vi "Rinocloud_get_metadata_field_value.vi"(6 "id":string, 9 "JSON Tree Expanded Reference":refnum<vi>) -> (0 "Notes":string, 1 "Tags":string, 2 "Name":string, 3 "Tree Ref out":refnum<vi>, 4 "body":string, 5 "headers":string)   [LabVIEW 2013]
uses:
  Rinocloud_global_variable.vi
  <vilib>/httpClient/POSTBuffer.vi
  <vilib>/LVH/i3 JSON/JSON Parsing/Get Object Parameter Files/Get Object Parameter - String.vi
  <vilib>/LVH/i3 JSON/JSON Parsing/Get Object Parameter Files/Get Object Parameter - Array.vi
  <vilib>/LVH/i3 JSON/JSON Parsing/Get Array Value at Index Files/Get Array Value at Index - String.vi
  <vilib>/httpClient/LabVIEWHTTPClient.lvlib
  i3 JSON/i3-json.lvlib
panel:
  out "JSON Tree":variant
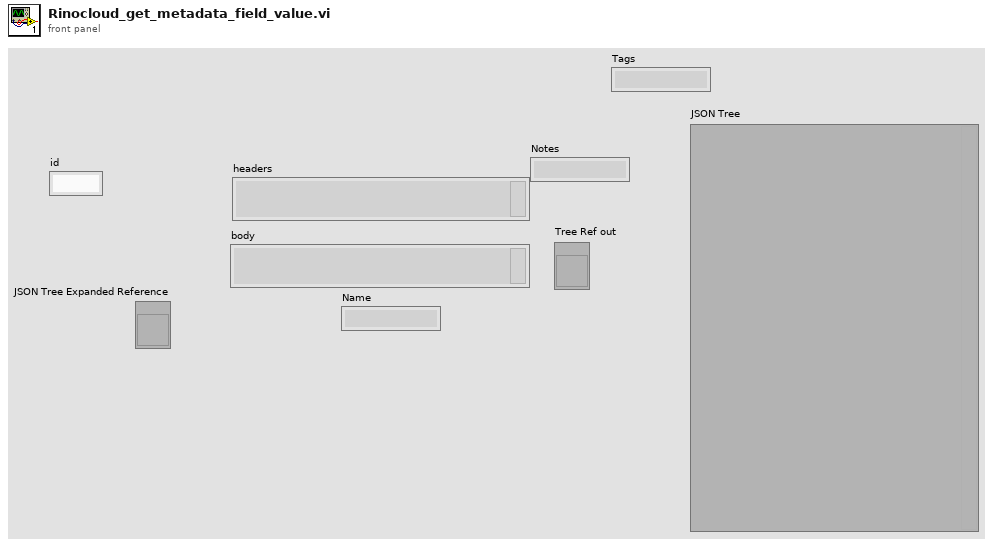
[diagram p1: front panel]
types:
  T1 = typedef "LabVIEWHTTPClient.lvlib/ClientHandle.ctl" = refnum<k1>
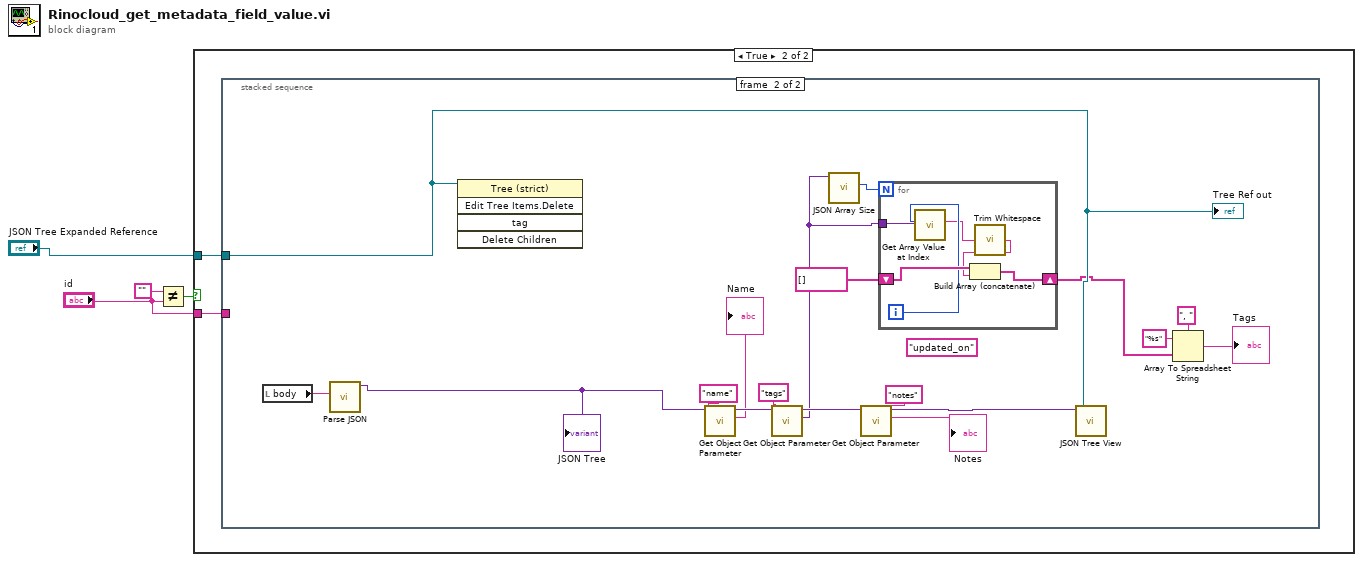
[diagram p0: block diagram]
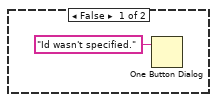
[diagram p2: hidden frame]
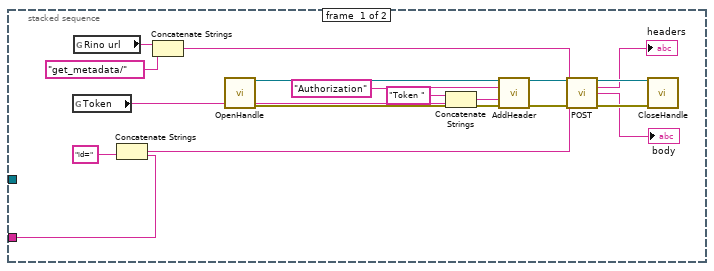
[diagram p3: hidden frame]
diagram:
  n1 = Not Equal?(x="", y="id") -> (x != y?=w3:bool)
  n2 = case shown="True" w3 {
    tunnel: "JSON Tree Expanded Reference" -> [_ w7]
    tunnel: "id" -> [_ w6]
    frame False {
      n3 = One Button Dialog(message="Id wasn't specified.") -> ()  [unwired: 1 in, 1 out]
    }
    frame True {
      n4 = stacked-sequence {
        tunnel: w7 -> [_ w34]
        tunnel: w6 -> [w9 _]
        frame #0 {
          n5 = global read "Rinocloud_global_variable.vi" "Token"() -> (w17:string)
          n6 = global read "Rinocloud_global_variable.vi" "Rino url"() -> (w23:string)
          n7 = Concatenate Strings("id=" ("value"), w9) -> (w8:string)
          n8 = Concatenate Strings(w23, "get_metadata/" ("Combo Box 2")) -> (w25:string)
          n9 = call <vilib>:"OpenHandle.vi"() -> ("client handle out"=w21:T1, "error out"=w18:errorcluster)  [unwired: 14 in]
          n10 = Concatenate Strings("Token " ("value"), w17) -> (w19:string)
          n11 = call <vilib>:"AddHeader.vi"("client handle"=w21, "header"="Authorization" ("url"), "value"=w19, "error in (no error)"=w18) -> ("client handle out"=w14:T1, "error out"=w13:errorcluster)  [unwired: 10 in]
          n12 = call-poly <vilib>:"POST.vi"("client handle"=w14, "url"=w25, "buffer"=w8, "error in (no error)"=w13) -> ("client handle out"=w16:T1, "headers"=→"headers":string, "body"=→"body":string, "error out"=w15:errorcluster)  [unwired: 8 in]
          n13 = call <vilib>:"CloseHandle.vi"("client handle"=w16, "error in (no error)"=w15) -> ()  [unwired: 13 in, 1 out]
        }
        frame #1 {
          (unwired) "updated_on" ("Parameter Name")
          n14 = local read "body"() -> (w43:string)
          n15 = call <vilib>:"Parse JSON.vi"("JSON String"=w43) -> ("JSON Tree"=w33:variant)  [unwired: 7 in, 3 out]
          "JSON Tree" <- w33
          n16 = invoke class="Tree (strict)" method="Edit Tree Items.Delete"(reference=w34) -> ()  [unwired: 4 in, 5 out]
          n17 = call-poly <vilib>:"Get Object Parameter.vi"("Parameter Name"="name", "JSON Tree In (JSON Object)"=w33) -> ("String Value"=→"Name":string, "JSON Tree Out Passthrough"=w40:variant)  [unwired: 6 in, 2 out]
          n18 = call-poly <vilib>:"Get Object Parameter.vi"("Parameter Name"="tags", "JSON Tree In (JSON Object)"=w40) -> ("JSON Array"=w31:variant, "JSON Tree Out Passthrough"=w38:variant)  [unwired: 6 in, 2 out]
          n19 = call <vilib>:"JSON Array Size.vi"("JSON Tree In (JSON Array)"=w31) -> ("Array Size"=w32:i32)  [unwired: 8 in, 2 out]
          n20 = call-poly <vilib>:"Get Object Parameter.vi"("Parameter Name"="notes", "JSON Tree In (JSON Object)"=w38) -> ("String Value"=→"Notes":string, "JSON Tree Out Passthrough"=w35:variant)  [unwired: 6 in, 2 out]
          n21 = for {
            N: w32 -> [_]
            tunnel: w31 -> [w49]
            shift-right: [w47] -> w27
            shift-left: string[] [] ("Tags 2") -> [w48]
            i -> [w46]
            n22 = call-poly <vilib>:"Get Array Value at Index.vi"("Index"=w46, "JSON Tree In (JSON Array)"=w49) -> ("String Value"=w45:string)  [unwired: 6 in, 3 out]
            n23 = call <vilib>:"Trim Whitespace.vi"("string"=w45) -> ("trimmed string"=w44:string)  [unwired: 1 in]
            n24 = Build Array (concatenate)(w48, w44) -> (w47:string[])
          }
          n25 = call "JSON Tree View.vi"("JSON Tree Expanded Reference"=w34, "JSON Tree"=w35) -> ()  [unwired: 8 in, 2 out]
          n26 = Array To Spreadsheet String(delimiter (Tab)=", ", array=w27, 3:"%s" ("format string")) -> (spreadsheet string=→"Tags":string)
          "Tree Ref out" <- w34
        }
      }
    }
  }
